vi "Scene List.vi"(8 "error in (no error)":errorcluster, 11 "OBS in":refnum<class "OBS.lvclass">) -> (0 "error out":errorcluster, 1 "Preview Scene":string, 2 "Program Scene":string, 3 "OBS out":refnum<class "OBS.lvclass">, 4 "Scenes":T1[](array[typedef]))   [LabVIEW 2022 SP3, in "obs-websocket-lv.lvlib" / "OBS.lvclass"]
uses:
  OBS.lvclass
  OBS.lvclass/OBS.ctl
  GetSceneList/GetSceneList.lvclass
  RGetSceneList/RGetSceneList.lvclass
  C:/dev/illuminatedg/obs-websocket-lv/obs-websocket-lv/Response/Response.lvclass
  C:/dev/illuminatedg/obs-websocket-lv/obs-websocket-lv/Server Message/Server Message.lvclass
  C:/dev/illuminatedg/obs-websocket-lv/obs-websocket-lv/Message/Message.lvclass
  C:/dev/illuminatedg/obs-websocket-lv/obs-websocket-lv/RGetSceneList/RGetSceneList.lvclass
  C:/dev/illuminatedg/obs-websocket-lv/obs-websocket-lv/Request/Request.lvclass
  C:/dev/illuminatedg/obs-websocket-lv/obs-websocket-lv/Client Message/Client Message.lvclass
  C:/dev/illuminatedg/obs-websocket-lv/obs-websocket-lv/GetSceneList/GetSceneList.lvclass
  Scene.ctl
  obs-websocket-lv.lvlib
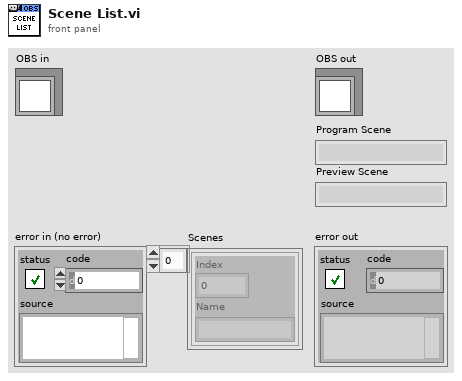
[diagram p1: front panel]
types:
  T1 = typedef "obs-websocket-lv.lvlib/Scene.ctl" = cluster{"Index":i32, "Name":string}
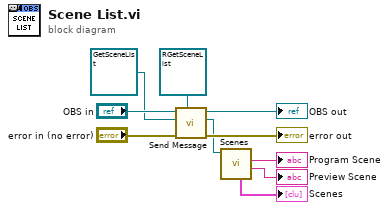
[diagram p0: block diagram]
diagram:
  n1 = call "Send Message.vi"("Response Type (None)"=refnum<class "RGetSceneList.lvclass"> refnum ("obs-websocket-lv.lvlib:RGetSceneList.lvclass"), "error in (no error)"="error in (no error)", "Client Message"=refnum<class "GetSceneList.lvclass"> refnum ("obs-websocket-lv.lvlib:GetSceneList.lvclass"), "OBS in"="OBS in") -> ("error out"=→"error out":errorcluster, "Response"=w1:refnum<class "RGetSceneList.lvclass">, "OBS out"=→"OBS out":refnum<class "OBS.lvclass">)  [unwired: 4 in, 1 out]
  n2 = call "Scenes.vi"("RGetSceneList in"=w1) -> ("Preview Scene"=→"Preview Scene":string, "Program Scene"=→"Program Scene":string, "Scenes"=→"Scenes":T1[])  [unwired: 6 in, 2 out]
